vi "_SubVI.vi"(1 "Closeable?":bool=TRUE, 3 "Type":T1=enum."Timer Window") -> ()   [LabVIEW 2014, in "UI_ProgressDlg.lvlib"]
uses:
  UI_ProgressDlg.lvlib
  _Control/DEF-Type.ctl
  UI_ProgressDlg.lvclass
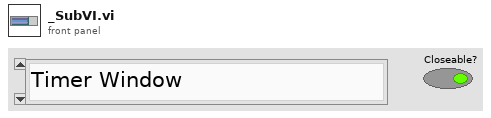
[diagram p1: front panel]
types:
  T1 = typedef "UI_ProgressDlg.lvlib/UI_ProgressDlg.lvclass/DEF-Type.ctl" = enum16{"Progress Window", "Buzy Window", "Timer Window"}
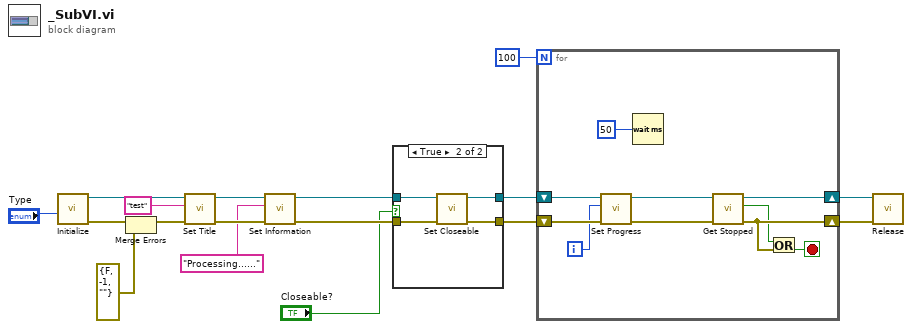
[diagram p0: block diagram]
diagram:
  n1 = call "Initialize.vi"("Type"="Type") -> ("error out"=w1:errorcluster, "UI_ProgressBar out"=w17:refnum<class "UI_ProgressDlg.lvclass">)  [unwired: 8 in, 1 out]
  n2 = Merge Errors(w1, errorcluster {"status"=FALSE, "code"=-1, "source"=""} ("error in")) -> (w7:errorcluster)
  n3 = call "Set Title.vi"("error in (no error)"=w7, "title"="test", "UI_ProgressBar in"=w17) -> ("error out"=w14:errorcluster, "UI_ProgressBar out"=w15:refnum<class "UI_ProgressDlg.lvclass">)  [unwired: 7 in]
  n4 = call "Set Information.vi"("error in (no error)"=w14, "Inforamtion"="Processing......", "UI_ProgressBar in"=w15) -> ("error out"=w4:errorcluster, "UI_ProgressBar out"=w12:refnum<class "UI_ProgressDlg.lvclass">)  [unwired: 7 in]
  n5 = case shown="True" "Closeable?" {
    tunnel: w12 -> [w19 w23]
    tunnel: [w19 w22] -> w5
    tunnel: w4 -> [w18 w21]
    tunnel: [w18 w20] -> w3
    frame False {
    }
    frame True {
      n6 = call "Set Closeable.vi"("error in (no error)"=w21, "UI_ProgressBar in"=w23) -> ("error out"=w20:errorcluster, "UI_ProgressBar out"=w22:refnum<class "UI_ProgressDlg.lvclass">)  [unwired: 8 in]
    }
  }
  n7 = for {
    N: 100 -> [_]
    shift-right: [w28] -> w11
    shift-left: w5 -> [w33]
    shift-right: [w26] -> w10
    shift-left: w3 -> [w31]
    i -> [w30]
    stop <- w25 stop-if-true
    n8 = call "Set Progress.vi"("error in (no error)"=w31, "progress"=w30, "UI_ProgressBar in"=w33) -> ("error out"=w27:errorcluster, "UI_ProgressBar out"=w32:refnum<class "UI_ProgressDlg.lvclass">)  [unwired: 7 in]
    n9 = Wait (ms)(milliseconds to wait=u32 50) -> ()  [unwired: 1 out]
    n10 = call "Get Stopped.vi"("error in (no error)"=w27, "UI_ProgressDlg in"=w32) -> ("error out"=w26:errorcluster, "Stopped?"=w24:bool, "UI_ProgressDlg out"=w28:refnum<class "UI_ProgressDlg.lvclass">)  [unwired: 7 in]
    n11 = Or(x=w24, y=w26) -> (x .or. y?=w25:bool)
  }
  n12 = call "Release.vi"("error in (no error)"=w10, "UI_ProgressBar in"=w11) -> ()  [unwired: 8 in, 2 out]
